vi "Find Hook.vi"(7 "Search Path":path[](array[path]), 8 "Error In":errorcluster, 11 "Hook":T1=enum."Pre-Dig") -> (0 "Error Out":errorcluster, 3 "Hook":path)   [LabVIEW 2018, in "Toolkit.lvlib"]
uses:
  Toolkit.lvlib
  Typedefs/Hooks.ctl
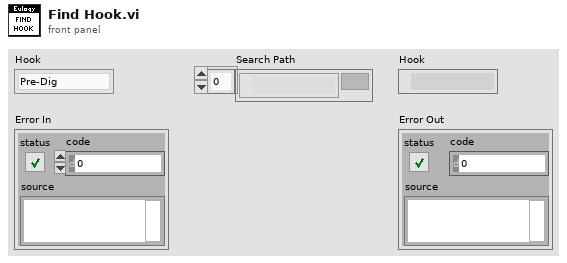
[diagram p1: front panel]
types:
  T1 = typedef "Toolkit.lvlib/Hooks.ctl" = enum16{"Pre-Bury", "Post-Bury", "Pre-Dig", "Post-Dig", "Pre-Reanimate", "Post-Reanimate", "Pre-Smite", "Post-Smite"}
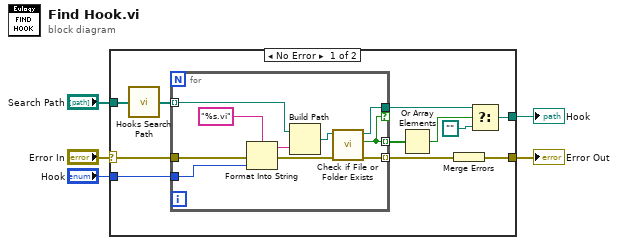
[diagram p0: block diagram]
diagram:
  n1 = case shown="No Error" "Error In" {
    selector: "Error In" -> [w13 w27]
    tunnel: "Hook" -> [w16 _]
    tunnel: [w9 _] -> w4
    tunnel: [w14 w27] -> w3
    tunnel: "Search Path" -> [w7 _]
    frame No Error {
      n2 = call "Hooks Search Path.vi"("Additional Search Path"=w7) -> ("Hooks Search Path"=w6:path[])
      n3 = for {
        tunnel: w16 -> [w25]
        tunnel: w13 -> [w24]
        tunnel: [w20] -> w10 if=w18
        tunnel: [w19] -> w15 mode=indexing
        tunnel: [w18] -> w12 mode=indexing
        tunnel: w6 -> [w17] mode=indexing
        n4 = Format Into String(format string="%s.vi", error in=w24, w25) -> (resulting string=w23:string, error out=w21:errorcluster)  [unwired: 1 in]
        n5 = Build Path(base path=w17, name or relative path=w23) -> (appended path=w22:path)
        n6 = call <vilib>:"Check if File or Folder Exists.vi"("error in (no error)"=w21, "path"=w22) -> ("error out"=w19:errorcluster, "file or folder exists?"=w18:bool, "dup path"=w20:path)  [unwired: 7 in]
      }
      n7 = Or Array Elements(Boolean array=w12) -> (logical OR=w11:bool)
      n8 = Merge Errors(w15) -> (w14:errorcluster)
      n9 = Select(t=w10, s=w11, f=path "") -> (s? t:f=w9:path)
    }
    frame Error {
    }
  }
  "Hook" <- w4
  "Error Out" <- w3
